vi "Agilent VNA Read External Trigger Mode.vi"(7 "Agilent VNA":T1, 8 "error in (no error)":errorcluster, 11 "VISA Resource Name":refnum<visa-resource-name>) -> (0 "error out":errorcluster, 2 "Ext. Trigger Mode":T2, 3 "dup VISA Resource Name":refnum<visa-resource-name>)   [LabVIEW 2011]
doc: "This VI for the HP8753B Network Analyzers reads the stimulus values. Except when performing log sweeps and freq list sweeps, this VI uses the start and stop values and the number of points to calcuate the stimulus values."
uses:
  TypeDefs/Agilent VNA External Trigger Mode.ctl
  TypeDefs/Agilent VNA Instrument Info.ctl
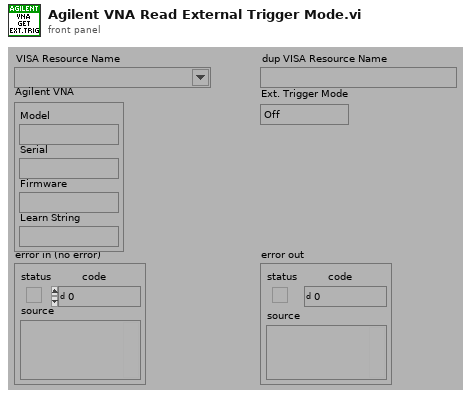
[diagram p1: front panel]
types:
  T1 = typedef "Agilent VNA Instrument Info.ctl" = cluster{"Model":string, "Serial":string, "Firmware":string, "Learn String":string}
  T2 = typedef "Agilent VNA External Trigger Mode.ctl" = enum16{"Off", "On Sweep", "On Point", "Manual On Point", "Internal", "External", "Bus"}
  T3 = typedef "Agilent VNA Model.ctl" = enum16{"Not Supported", "8510X", "8719X", "8720X", "8722X", "8753X", "ENA", "PNA", "Field Fox"}
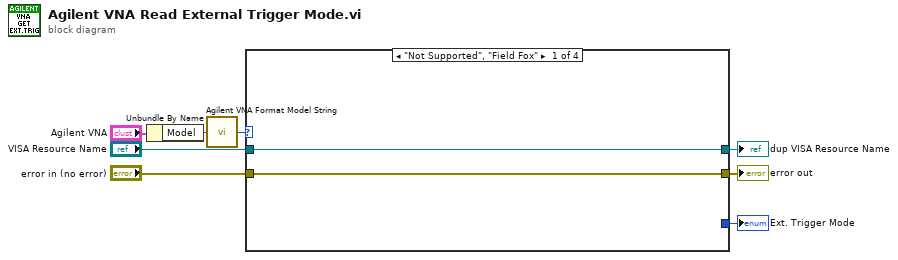
[diagram p0: block diagram]
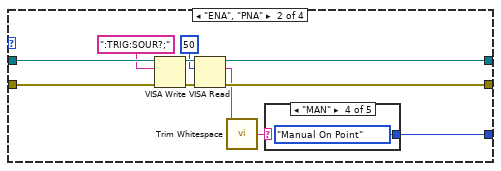
[diagram p2: hidden frame]
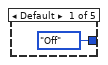
[diagram p3: hidden frame]
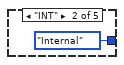
[diagram p4: hidden frame]
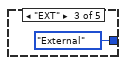
[diagram p5: hidden frame]
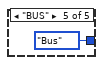
[diagram p6: hidden frame]
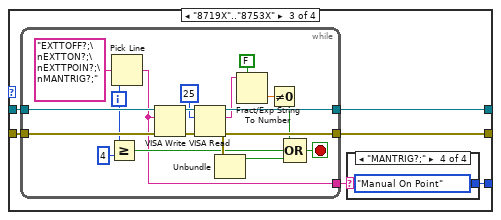
[diagram p7: hidden frame]
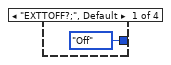
[diagram p8: hidden frame]
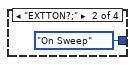
[diagram p9: hidden frame]
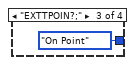
[diagram p10: hidden frame]
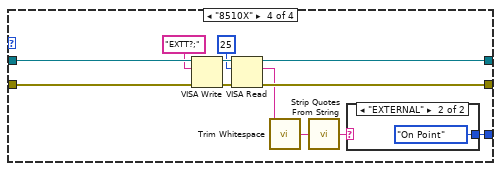
[diagram p11: hidden frame]
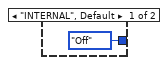
[diagram p12: hidden frame]
diagram:
  n1 = Unbundle By Name("Agilent VNA") -> ("Model"=w1:string)
  n2 = call "Agilent VNA Format Model String.vi"("Model"=w1) -> ("Model"=w3:T3)
  n3 = case shown="\"Not Supported\", \"Field Fox\"" w3 {
    tunnel: "error in (no error)" -> [w9 w17 w32 w66]
    tunnel: [w9 w16 w31 w65] -> w7
    tunnel: "VISA Resource Name" -> [w10 w18 w30 w64]
    tunnel: [w10 w15 w29 w63] -> w5
    tunnel: [_ w11 w28 w62] -> w4
    frame "Not Supported", "Field Fox" {
    }
    frame "ENA", "PNA" {
      n4 = VISA Write(VISA resource name=w18, write buffer=":TRIG:SOUR?;", error in (no error)=w17) -> (VISA resource name out=w21:refnum<visa-resource-name>, error out=w20:errorcluster)  [unwired: 1 out]
      n5 = VISA Read(VISA resource name=w21, byte count=u32 50, error in (no error)=w20) -> (VISA resource name out=w15:refnum<visa-resource-name>, read buffer=w13:string, error out=w16:errorcluster)  [unwired: 1 out]
      n6 = call <vilib>:"Trim Whitespace.vi"("string"=w13) -> ("trimmed string"=w12:string)  [unwired: 1 in]
      n7 = case shown="\"MAN\"" w12 {
        tunnel: [Agilent_VNA_External_Trigger_Mode."Off" Agilent_VNA_External_Trigger_Mode."Internal" Agilent_VNA_External_Trigger_Mode."External" Agilent_VNA_External_Trigger_Mode."Manual On Point" Agilent_VNA_External_Trigger_Mode."Bus"] -> w11
        frame Default {
        }
        frame "INT" {
        }
        frame "EXT" {
        }
        frame "MAN" {
        }
        frame "BUS" {
        }
      }
    }
    frame "8719X".."8753X" {
      n8 = while {
        tunnel: w32 -> [w54]
        tunnel: [w50] -> w31
        tunnel: w30 -> [w53]
        tunnel: [w49] -> w29
        tunnel: [w37] -> w27
        i -> [w43]
        stop <- w38 stop-if-true
        n9 = Greater Or Equal?(x=w43, y=4) -> (x >= y?=w39:bool)
        n10 = Pick Line(multi-line string="EXTTOFF?;\nEXTTON?;\nEXTTPOIN?;\nMANTRIG?;", line index=w43) -> (output string=w37:string)  [unwired: 1 out]
        n11 = VISA Write(VISA resource name=w53, write buffer=w37, error in (no error)=w54) -> (VISA resource name out=w52:refnum<visa-resource-name>, error out=w51:errorcluster)  [unwired: 1 out]
        n12 = VISA Read(VISA resource name=w52, byte count=u32 25, error in (no error)=w51) -> (VISA resource name out=w49:refnum<visa-resource-name>, read buffer=w46:string, error out=w50:errorcluster)  [unwired: 1 out]
        n13 = Unbundle(w50) -> ("status"=w40:bool)  [unwired: 2 out]
        n14 = Fract/Exp String To Number(use system decimal point (T)=FALSE, string=w46) -> (number=w44:dbl)  [unwired: 3 out]
        n15 = Not Equal To 0?(x=w44) -> (x != 0?=w41:bool)
        n16 = Compound Arithmetic op=OR(w41, w39, w40) -> (w38:bool)
      }
      n17 = case shown="\"MANTRIG?;\"" w27 {
        tunnel: [Agilent_VNA_External_Trigger_Mode."Off" Agilent_VNA_External_Trigger_Mode."On Sweep" Agilent_VNA_External_Trigger_Mode."On Point" Agilent_VNA_External_Trigger_Mode."Manual On Point"] -> w28
        frame "EXTTOFF?;", Default {
        }
        frame "EXTTON?;" {
        }
        frame "EXTTPOIN?;" {
        }
        frame "MANTRIG?;" {
        }
      }
    }
    frame "8510X" {
      n18 = VISA Write(VISA resource name=w64, write buffer="EXTT?;", error in (no error)=w66) -> (VISA resource name out=w61:refnum<visa-resource-name>, error out=w60:errorcluster)  [unwired: 1 out]
      n19 = VISA Read(VISA resource name=w61, byte count=u32 25, error in (no error)=w60) -> (VISA resource name out=w63:refnum<visa-resource-name>, read buffer=w56:string, error out=w65:errorcluster)  [unwired: 1 out]
      n20 = call <vilib>:"Trim Whitespace.vi"("string"=w56) -> ("trimmed string"=w57:string)  [unwired: 1 in]
      n21 = call "Strip Quotes From String.vi"("String In"=w57) -> ("Trimmed String"=w55:string)
      n22 = case shown="\"EXTERNAL\"" w55 {
        tunnel: [Agilent_VNA_External_Trigger_Mode."Off" Agilent_VNA_External_Trigger_Mode."On Point"] -> w62
        frame "INTERNAL", Default {
        }
        frame "EXTERNAL" {
        }
      }
    }
  }
  "dup VISA Resource Name" <- w5
  "error out" <- w7
  "Ext. Trigger Mode" <- w4
